vi "ExtractErrorInfo.vi"(11 "source in":string) -> (1 "result string":string, 2 "Callchain":string[](array[string]))   [LabVIEW 2024, in "DefaultLogFormat.lvclass"]
uses:
  DefaultLogFormat.lvclass
  <vilib>/Utility/error.llb/Trim Whitespace One-Sided.vi
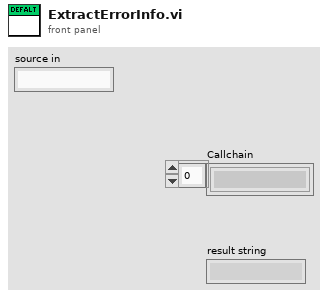
[diagram p1: front panel]
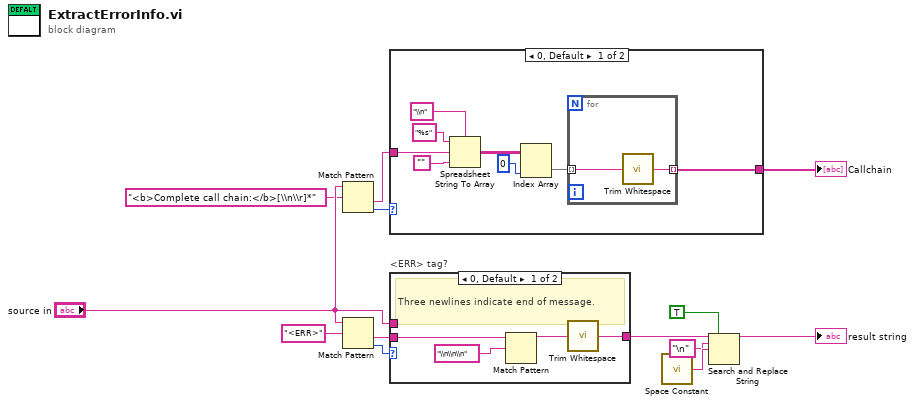
[diagram p0: block diagram]
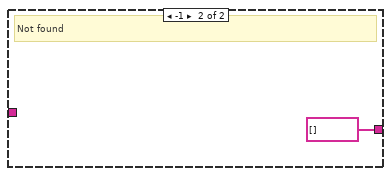
[diagram p3: hidden frame]
diagram:
  n1 = Match Pattern(string="source in", regular expression="<b>Complete call chain:</b>[\\n\\r]*") -> (after substring=w3:string, offset past match=w2:i32)  [unwired: 1 in, 2 out]
  n2 = Match Pattern(string="source in", regular expression="<ERR>") -> (after substring=w4:string, offset past match=w5:i32)  [unwired: 1 in, 2 out]
  n3 = case shown="0, Default" w2 {
    tunnel: [w14 string[] []] -> w13
    tunnel: w3 -> [w21 _]
    frame 0, Default {
      n4 = Spreadsheet String To Array(delimiter (Tab)="\\n", format string="%s", spreadsheet string=w21, array type (2D Dbl)="") -> (array=w18:string[][])
      n5 = Index Array(array=w18, index (col)=0 ("disabled index (col)")) -> (element=w15:string[])  [unwired: 1 in]
      n6 = for {
        tunnel: w15 -> [w23] mode=indexing
        tunnel: [w22] -> w14 mode=indexing
        n7 = call <vilib>:"Trim Whitespace.vi"("string"=w23) -> ("trimmed string"=w22:string)  [unwired: 1 in]
      }
    }
    frame -1 {
      # "Not found"
    }
  }
  "Callchain" <- w13
  n8 = case "<ERR> tag?" shown="0, Default" w5 {
    tunnel: w4 -> [w28 _]
    tunnel: "source in" -> [_ w29]
    tunnel: [w25 w29] -> w9
    frame 0, Default {
      # "Three newlines indicate end of message."
      n9 = Match Pattern(string=w28, regular expression="\\n\\n\\n") -> (before substring=w26:string)  [unwired: 1 in, 3 out]
      n10 = call <vilib>:"Trim Whitespace.vi"("string"=w26) -> ("trimmed string"=w25:string)  [unwired: 1 in]
    }
    frame -1 {
      # "No extended error information."
    }
  }
  n11 = call <vilib>:"Space Constant.vi"() -> ("String"=w10:string)
  n12 = Search and Replace String(replace all?=TRUE ("replace all? (F)"), input string=w9, search string="\n", replace string=w10) -> (result string=→"result string":string)  [unwired: 4 in, 3 out]
